vi "ke37xx Configure DAC-Totalizer Power State.vi"(8 "error in (no error)":errorcluster, 9 "Power State (True)":bool=TRUE, 10 "DAC/Totalizer Channel List":string, 11 "VISA Resource Name":refnum<visa-resource-name>) -> (0 "error out":errorcluster, 3 "VISA Resource Name Out":refnum<visa-resource-name>)   [LabVIEW 2009, in "Keithley 3700 Series.lvlib"]
doc: "This VI allows powering up/down of the Totalizer section of Digital I/O cards."
uses:
  <instrlib>/Keithley 3706/Keithley 3700 Series.lvlib
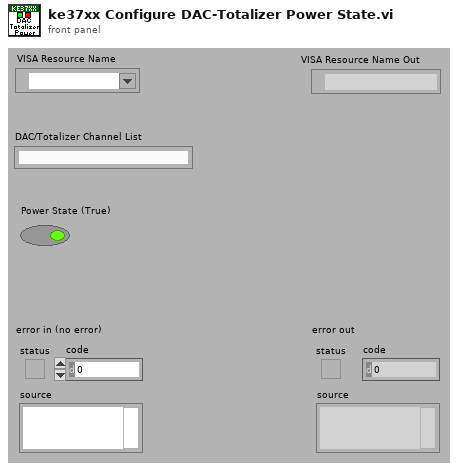
[diagram p1: front panel]
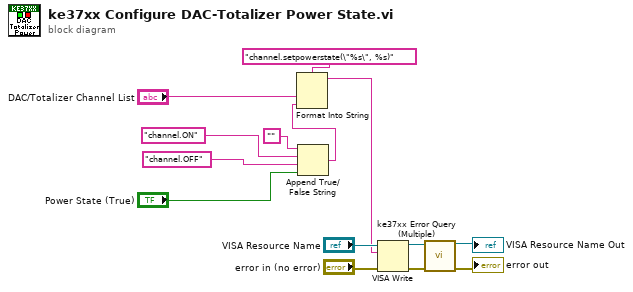
[diagram p0: block diagram]
diagram:
  n1 = Append True/False String(1:"Power State (True)", 2:"channel.OFF", 3:"channel.ON", 4:"") -> (0:w5:string)
  n2 = Format Into String(format string="channel.setpowerstate(\"%s\", %s)", "DAC/Totalizer Channel List", w5) -> (resulting string=w9:string)  [unwired: 2 in, 1 out]
  n3 = VISA Write(VISA resource name="VISA Resource Name", write buffer=w9, error in (no error)="error in (no error)") -> (VISA resource name out=w8:refnum<visa-resource-name>, error out=w7:errorcluster)  [unwired: 1 out]
  n4 = call <instrlib>:"ke37xx Error Query (Multiple).vi"("VISA resource name"=w8, "error in (no error)"=w7) -> ("VISA resource name out"=→"VISA Resource Name Out":refnum<visa-resource-name>, "error out"=→"error out":errorcluster)  [unwired: 12 out]
